vi "Read Post-Measurement Settling Cycles.vi"(8 "error in (no error)":errorcluster, 11 "signal configuration":refnum<class "SV Function.lvclass">) -> (0 "error out":errorcluster, 2 "post-measurement settling cycles":dbl, 3 "signal configuration":refnum<class "SV Function.lvclass">)   [LabVIEW 2017, in "SV Function.lvclass"]
uses:
  <vilib>/addons/_NISVFA/_Generation/Signal Generation/SV Function/SV Function.lvclass
  <vilib>/addons/_NISVFA/_Generation/Signal Generation/SV Function/SV Function.lvclass/SV Function.ctl
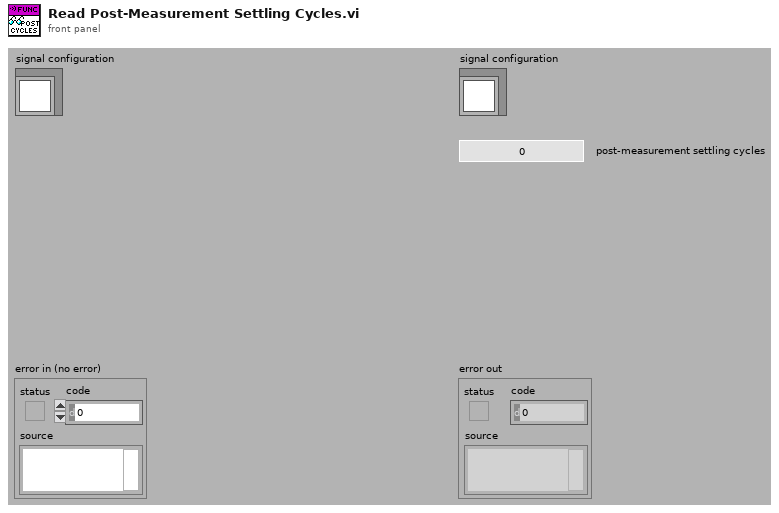
[diagram p1: front panel]
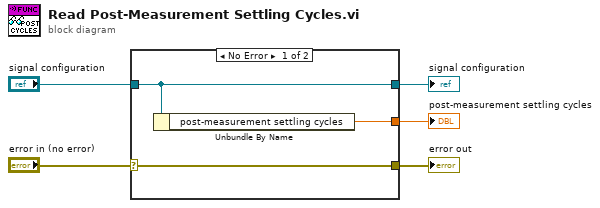
[diagram p0: block diagram]
diagram:
  n1 = case shown="No Error" "error in (no error)" {
    selector: "error in (no error)" -> [w8 w9]
    tunnel: [w8 w9] -> w4
    tunnel: [w7 w10] -> w2
    tunnel: "signal configuration" -> [w7 w10]
    tunnel: [w6 _] -> w1
    frame No Error {
      n2 = Unbundle By Name(w7) -> ("post-measurement settling cycles"=w6:dbl)
    }
    frame Error {
    }
  }
  "error out" <- w4
  "signal configuration" <- w2
  "post-measurement settling cycles" <- w1
